vi "Initial Values-Unbundler-Bool.vi"(8 "error in (no error)":errorcluster, 9 "Keys Array":T2, 10 "Section name":string, 11 "User profile ini file ref":T1) -> (0 "error out":errorcluster, 3 "User profile ini file ref":T1)   [LabVIEW 2020]
uses:
  Typedefs/Ini file interface (Boolean).ctl
  <vilib>/Utility/config.llb/Config Data RefNum.ctl
  Typedefs/HW config states enum.ctl
  Typedefs/Read Write Enum.ctl
  Global Variables/General Globals.vi
  Global Variables/gl_UI Ctrl Refs.vi
  <vilib>/Utility/config.llb/NI_LVConfig.lvlib
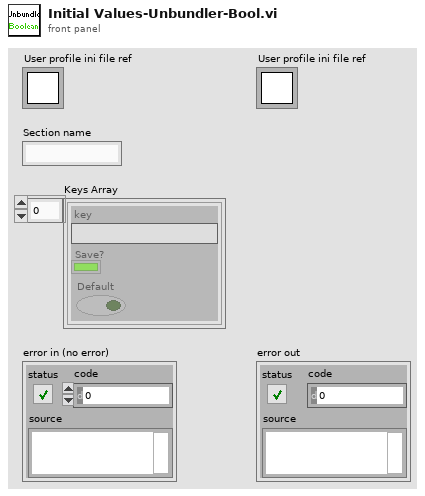
[diagram p1: front panel]
types:
  T1 = typedef "NI_LVConfig.lvlib/Config Data RefNum.ctl" = refnum<k1>
  T2 = typedef "Ini file interface (Boolean).ctl" = cluster{"key":string, "Save?":bool, "Default":bool}[]
  T3 = typedef "Read Write Enum.ctl" = enum16{"Read", "Write"}
  T4 = typedef "HW config states enum.ctl" = enum16{"Load from file", "Save to file", "Save backup", "Write all", "Read all", "Write XY stage settings", "Write DAQ FPGA settings", "Write Control FPGA settings", "Write Phys Channels", "Write System Config", "Write HW Config", "Save System Config", "Save HW Config", "Clear", "Compare from file"}
  T5 = typedef "Hardware Configuration settings.ctl" = cluster{"Dev. PC":bool, "Swap XY on stage":bool, "No of AOD":u8, "MC Supported":bool, "Axial MC":bool, "Computer MAC address":string, "Externalise Triggers":bool, "Trigger HW config":T6, "DAQmx Chan":T7, "XY stage available":bool, "XY Stage":T8, "Z stage available":bool, "Z Stage config cluster":T9, "Encoder available":bool, "Encoder":T10, "VidRec available":bool, "Cam VidRec":T11, "Laser Power Control HW config":T12, "Laser 1 available":bool, "Laser 1 config cluster":T13, "Prechirper 1 available":bool, "Prechirper 1 config cluster":T14, "Control system.FPGA available?":bool, "Control Sys. HW config":T15, "DAQ FPGA HW Config":T16, "PMT Voltage Range":T20}
  T6 = typedef "Triggers HW config.ctl" = cluster{"Available Device List":i32, "Device Address":string}
  T7 = typedef "DAQmx physical channels cluster.ctl" = cluster{"Pockels AO":tag, "Hard shutter AO":tag, "PMT AOs":tag, "Galvo AOs":tag, "Power meter AI":tag}
  T8 = typedef "XY Stage config cluster.ctl" = cluster{"COM port":refnum<visa-resource-name>, "Baudrate":i32, "Type":string}
  T9 = typedef "Z Stage config cluster.ctl" = cluster{"COM port":refnum<visa-resource-name>, "Baudrate":i32, "Type":string}
  T10 = typedef "Encoder config cluster.ctl" = cluster{"IP address":string, "Port":u16, "Wheel radius (cm)":dbl, "Encoder Trigger":tag}
  T11 = typedef "Cam VidRec HW config setup cluster.ctl" = cluster{"DO flag-Video record":tag, "DO flag-Trial start":tag}
  T12 = typedef "Laser Power Control HW config.ctl" = cluster{"Laser Power Control":string, "Laser Power Modulation Control":enum16{"NI", "FPGA"}}
  T13 = typedef "Laser 1 config cluster.ctl" = cluster{"COM port":refnum<visa-resource-name>, "Baud Rate":i32, "Type":string}
  T14 = typedef "PreChirper 1 config cluster.ctl" = cluster{"Type":string, "Baud Rate":i32, "COM port":refnum<visa-resource-name>}
  T15 = typedef "Control Sys HW config cluster.ctl" = cluster{"Control system.FPGA Type":enum16{"Virtex 5", "Virtex 7"}, "Control system.Network adapter name":string, "Control system.MAC address":string, "Control system.Ethernet Port":u32, "Control system.Ethernet Port Opened":bool}
  T16 = typedef "DAQ FPGA HW config cluster.ctl" = cluster{"FGPA Ref":T17, "Target":T18, "input card type":T19}
  T17 = typedef "FPGA Ref.ctl" = refnum<k20>
  T18 = typedef "nirio_resource_hc.ctl" = tag
  T19 = typedef "FPGA input type AC-DC.ctl" = enum16{"AC Card", "DC Card"}
  T20 = typedef "PMT Voltage Range.ctl" = cluster{"PMT Voltage Lower Limit":dbl, "PMT Voltage Upper Limit":dbl}
  T21 = typedef "UI ctrl refs cluster.ctl" = cluster{"Top level VI path":path, "Top level VI ref":refnum<vi>, "User menu ref":refnum<k9>, "Sub Panel control":refnum<vi>, "Imaging Param Tab":refnum<vi>, "Occurrence-Start drivers":refnum<k4>, "Occurrence-Speed logging initialised":refnum<k4>, "Occurrence-XYZ stage initialised":refnum<k4>, "Exit button":refnum<vi>, "Status ind":refnum<vi>, "Set as origin":refnum<vi>, "Speed Logging":refnum<vi>, "Time Lapse":refnum<vi>, "Live Imaging":refnum<vi>, "AOL Z Stack":refnum<vi>, "Motor Z Stack":refnum<vi>, "Funct Acq button":refnum<vi>, "Hard Shutter":refnum<vi>, "Virtual Shutter":refnum<vi>, "Laser Power":refnum<vi>, "AOL Mode":refnum<vi>, "Frame Size":refnum<vi>, "Field of View":refnum<vi>, "Dwell Time":refnum<vi>, "Zoom":refnum<vi>, "AOL Z":refnum<vi>, "Objective":refnum<vi>, "Axis":refnum<vi>, "Paths & Names":refnum<vi>, "Experiment folder path (ind.)":refnum<vi>, "Last State (Ind.)":refnum<vi>, "Averages":refnum<vi>, "Angle (degrees)":refnum<vi>, "X centre":refnum<vi>, "Y centre":refnum<vi>, "Plane Mode":refnum<vi>, "# Planes":refnum<vi>, "Z Start":refnum<vi>, "Z Stop":refnum<vi>, "Z Step":refnum<vi>, "PMT 1":refnum<vi>, "PMT 2":refnum<vi>, "Stage XYZ Position":refnum<vi>, "Pockels@Z Start":refnum<vi>, "Pockels@Z Stop":refnum<vi>, "Obtain Z Start":refnum<vi>, "Obtain Z Stop":refnum<vi>, "Live stim.trig.period":refnum<vi>, "Live stim.trig.enable":refnum<vi>, "Movement Correction":refnum<vi>, "Load Reference Image":refnum<vi>, "XY Stage Move":refnum<vi>, "MovCor Cluster":refnum<vi>, "RefDAQParam":refnum<vi>, "Funct. Acq. Pockels Modulation":refnum<vi>, "Ref Laser Power":refnum<vi>, "Enable Video Recording":refnum<vi>, "Video Record-Live Imaging":refnum<vi>, "Video Record-Funct acq":refnum<vi>, "Reference Source":refnum<vi>, "AOL Z-stack Chirps Ready (ind)":refnum<vi>, "Target time between mov.cor. ref triggers (ms)":refnum<vi>, "Funct. Acq. Ref frame save":refnum<vi>, "Tracking button":refnum<vi>, "Show ref plots window":refnum<vi>, "Center freq ind (nm)":refnum<vi>, "Pickup mode (ind)":refnum<vi>, "Logging queue (ind)":refnum<vi>, "Back aperture power (ind.)":refnum<vi>, "Power after objective (ind.)":refnum<vi>, "Switch user":refnum<vi>, "Ls1 Conn. Status":refnum<vi>, "Ls1Tuning Status":refnum<vi>, "Ls1 Faults":refnum<vi>, "Ls1 Connection":refnum<vi>, "Ls1 Mode":refnum<vi>, "Ls1 POWER [mW]":refnum<vi>, "Ls1Shutter":refnum<vi>, "Ls1 Wavelength":refnum<vi>, "Ls1 Note":refnum<vi>, "Ls1 Confirm Wav":refnum<vi>, "Ls1 PreChrp Prism1":refnum<vi>, "Ls1 PreChrp Prism2":refnum<vi>, "Ls1 wav top Ind":refnum<vi>, "Ls1 power top Ind":refnum<vi>, "Ls1 Pump peak Hold":refnum<vi>, "Ls1 Status Ind":refnum<vi>, "Ls1 wav cancel":refnum<vi>, "Experiment Type":refnum<vi>, "Biology Information":refnum<vi>, "Camera recording status":refnum<vi>}
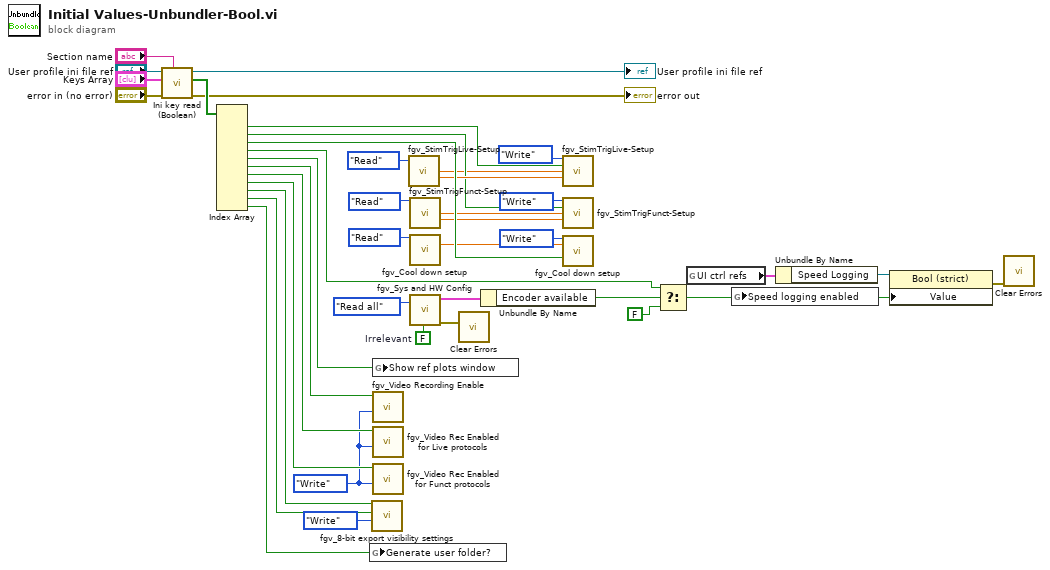
[diagram p0: block diagram]
diagram:
  w1 = FALSE  # Irrelevant
  w9 = Read_Write_Enum."Write" ("Function")
  n1 = call "Ini key read (Boolean).vi"("Section"="Section name", "error in (no error)"="error in (no error)", "Parameter names & setup"="Keys Array", "Ini file refnum in"="User profile ini file ref") -> ("error out"=→"error out":errorcluster, "Value read/used"=w27:bool[], "Ini file refnum out"=→"User profile ini file ref":T1)  [unwired: 5 in]
  n2 = Index Array(array=w27) -> (element #1=w31:bool, element #2=w35:bool, element #3=w41:bool, element #4=w15:bool, element #5=w13:bool, element #6=w12:bool, element #7=w11:bool, element #8=w10:bool, element #9=w7:bool, element #10=w6:bool, element #11=w3:bool)  [unwired: 11 in]
  n3 = global write "General Globals.vi" "Generate user folder?"(w3) -> ()
  n4 = call "fgv_8-bit export visibility settings.vi"("Function"=enum16{"Intialize", "Write", "Read", "Clear"}."Write", "Include camera videos"=w6, "Include speed graph"=w7) -> ()  [unwired: 6 in, 3 out]
  n5 = global write "General Globals.vi" "Show ref plots window"(w13) -> ()
  n6 = call "fgv_Video Recording Enable.vi"("Function"=w9, "Video Recording Enabled"=w12) -> ()  [unwired: 8 in, 2 out]
  n7 = call "fgv_Video Rec Enabled for Live protocols.vi"("Function"=w9, "Video Recording Enabled for Live protocols"=w11) -> ()  [unwired: 9 in, 1 out]
  n8 = call "fgv_Video Rec Enabled for Funct protocols.vi"("Function"=w9, "Video Recording Enabled for functional acq protocols"=w10) -> ()  [unwired: 9 in, 1 out]
  n9 = call "fgv_StimTrigLive-Setup.vi"("Function"=enum16{"Intialize", "Write", "Read", "Clear"}."Read") -> ("Live stim.trig.period (sec)"=w30:dbl, "Live stim.trig.width (ms)"=w36:dbl)  [unwired: 11 in, 2 out]
  n10 = call "fgv_StimTrigFunct-Setup.vi"("Function"=enum16{"Intialize", "Write", "Read", "Clear"}."Read") -> ("Funct stim.trig.delay (sec)"=w37:dbl, "Funct stim.trig.width (ms)"=w34:dbl)  [unwired: 11 in, 2 out]
  n11 = call "fgv_Cool down setup.vi"("Function"=enum16{"Intialize", "Write", "Read", "Clear"}."Read") -> ("Cool-down time (s)"=w40:dbl)  [unwired: 12 in, 2 out]
  n12 = call "fgv_Sys and HW Config.vi"("Standalone viewer initialisation?"=w1, "Function"=HW_config_states_enum."Read all") -> ("error out"=w2:errorcluster, "Hardware Configuration OUT"=w20:T5)  [unwired: 7 in, 1 out]
  n13 = call <vilib>:"Clear Errors.vi"("error in (no error)"=w2) -> ()  [unwired: 5 in, 2 out]
  n14 = Unbundle By Name(w20) -> ("Encoder available"=w16:bool)
  n15 = call "fgv_StimTrigLive-Setup.vi"("Function"=enum16{"Intialize", "Write", "Read", "Clear"}."Write", "Live stim.trig.enable"=w31, "Live stim.trig.period (sec)"=w30, "Live stim.trig.width (ms)"=w36) -> ()  [unwired: 8 in, 4 out]
  n16 = call "fgv_StimTrigFunct-Setup.vi"("Function"=enum16{"Intialize", "Write", "Read", "Clear"}."Write", "Funct stim.trig.enable"=w35, "Funct stim.trig.delay (sec)"=w37, "Funct stim.trig.width (ms)"=w34) -> ()  [unwired: 8 in, 4 out]
  n17 = call "fgv_Cool down setup.vi"("Function"=enum16{"Intialize", "Write", "Read", "Clear"}."Write", "Cool-down time (s)"=w40, "Enable cool-down time"=w41) -> ()  [unwired: 10 in, 3 out]
  n18 = Select(t=w15, s=w16, f=FALSE) -> (s? t:f=w5:bool)
  n19 = global read "gl_UI Ctrl Refs.vi" "UI ctrl refs"() -> (w17:T21)
  n20 = global write "General Globals.vi" "Speed logging enabled"(w5) -> ()
  n21 = Unbundle By Name(w17) -> ("Speed Logging"=w18:refnum<vi>)
  n22 = property class="Bool (strict)"(reference=w18, "Value"=w5) -> (error out=w4:errorcluster)  [unwired: 1 in, 1 out]
  n23 = call <vilib>:"Clear Errors.vi"("error in (no error)"=w4) -> ()  [unwired: 5 in, 2 out]
